vi "Parametric Tester.vi"() -> ()   [LabVIEW 2017]
uses:
  <vilib>/Utility/file.llb/Write To Spreadsheet File (string).vi
  <vilib>/Utility/file.llb/Write To Spreadsheet File (DBL).vi
panel:
  in  "Header Info":string[][](table)=[["Test Name", "Operator", "UUT"], ["Voltage Test", "Nigel", "AAA123"]]
  in  "File Name":path=path "C:/Documents and Settings/husmith/Desktop/CSVdata.csv"
  in  "Channel Names":string[](array[string])=["Channel 1", "Channel 2", "Channel 3", "Channel 4", "Channel 5"]
  in  "# of Channels":i32=5
  in  "stop":bool
  in  "Values to Write":i32=20
  out "Forearm\nAngle":dbl
  out "Backarm\nAngle":dbl
  in  "New Parametric\nValue":dbl
  in  "Points":dbl[][](array[numeric])
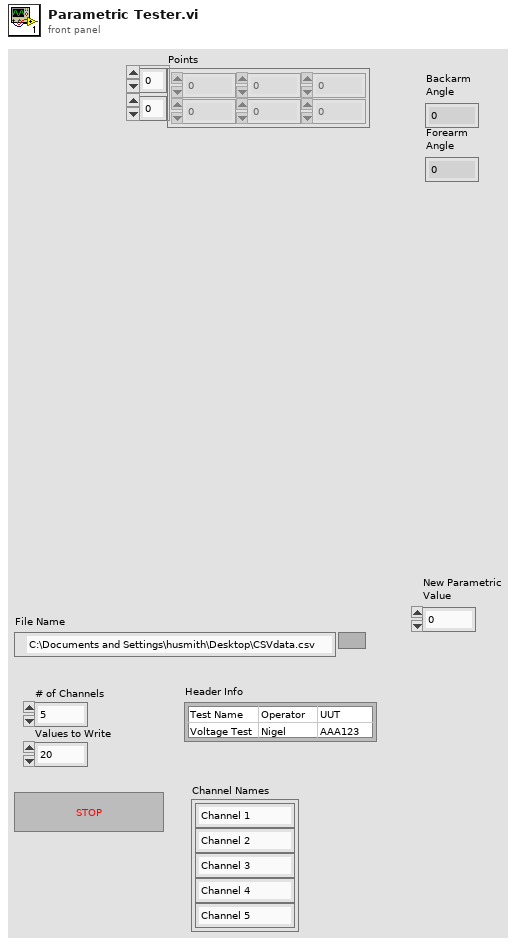
[diagram p1: front panel]
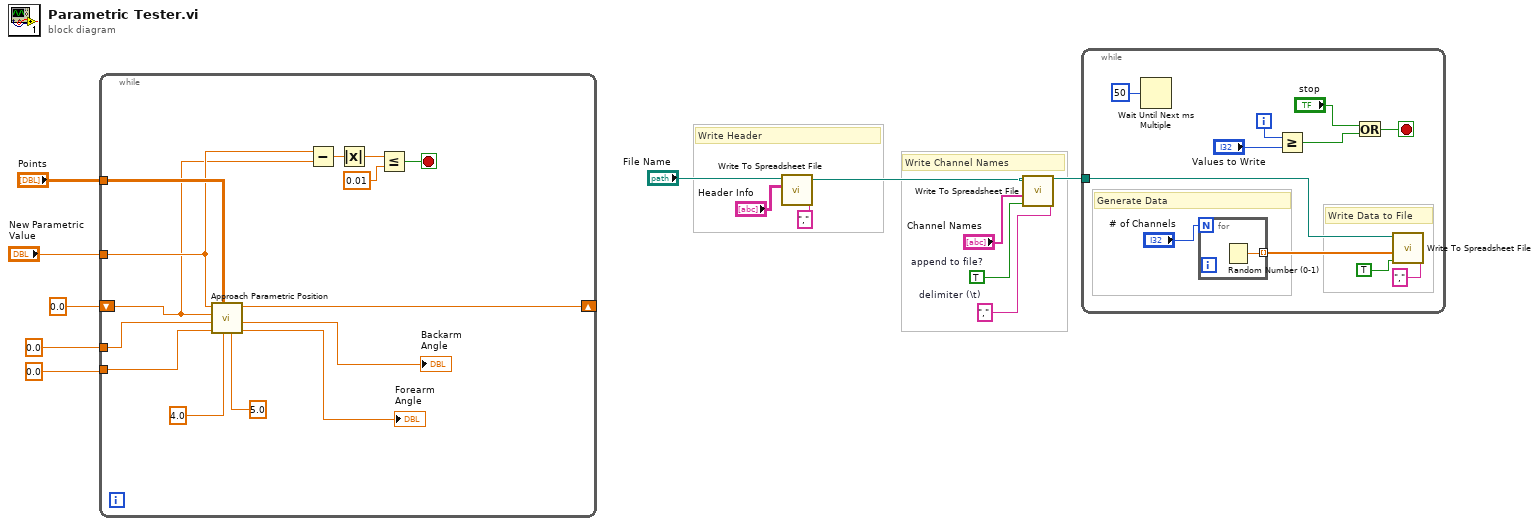
[diagram p0: block diagram]
diagram:
  w4 = TRUE  # append to file?
  w5 = ","  # delimiter (\t)
  # "Write Header"
  # "Write Channel Names"
  n1 = while {
    shift-right: [w23] -> _
    shift-left: 0.0 -> [w20]
    tunnel: "New Parametric\nValue" -> [w21]
    tunnel: 0.0 -> [w27]
    tunnel: 0.0 -> [w26]
    tunnel: "Points" -> [w22]
    stop <- w16 stop-if-true
    n2 = call "Approach Parametric Position.vi"("Forearm Length"=5.0, "Backarm Length"=4.0, "Points"=w22, "Initial Forearm\nAngle"=w26, "Initial Backarm\nAngle"=w27, "Initial Parametric\nValue"=w20, "New Parametric\nValue"=w21) -> ("Next Forearm\nAngle"=→"Forearm\nAngle":dbl, "Next Backarm\nAngle"=→"Backarm\nAngle":dbl, "Next Parametric\nValue"=w23:dbl)  [unwired: 2 in]
    n3 = Subtract(x=w21, y=w20) -> (x-y=w19:dbl)
    n4 = Absolute Value(x=w19) -> (abs(x)=w18:dbl)
    n5 = Less Or Equal?(x=w18, y=0.01) -> (x <= y?=w16:bool)
  }
  n6 = call-poly <vilib>:"Write To Spreadsheet File.vi"("delimiter (\\t)"="," ("delimiter (\\t)"), "2D data"="Header Info", "file path (dialog if empty)"="File Name") -> ("new file path (Not A Path if cancelled)"=w6:path)  [unwired: 4 in, 1 out]
  n7 = call-poly <vilib>:"Write To Spreadsheet File.vi"("delimiter (\\t)"=w5, "append to file? (new file:F)"=w4, "1D data"="Channel Names", "file path (dialog if empty)"=w6) -> ("new file path (Not A Path if cancelled)"=w8:path)  [unwired: 3 in, 1 out]
  n8 = while {
    tunnel: w8 -> [w30]
    i -> [w35]
    stop <- w32 stop-if-true
    # "Write Data to File"
    # "Generate Data"
    n9 = Wait Until Next ms Multiple(millisecond multiple=u32 50) -> ()  [unwired: 1 out]
    n10 = for {
      N: "# of Channels" -> [_]
      tunnel: [w39] -> w31 mode=indexing
      n11 = Random Number (0-1)() -> (number: 0 to 1=w39:dbl)
    }
    n12 = Greater Or Equal?(x=w35, y="Values to Write") -> (x >= y?=w33:bool)
    n13 = Or(x="stop", y=w33) -> (x .or. y?=w32:bool)
    n14 = call-poly <vilib>:"Write To Spreadsheet File.vi"("delimiter (\\t)"="," ("delimiter (\\t)"), "append to file? (new file:F)"=TRUE, "1D data"=w31, "file path (dialog if empty)"=w30) -> ()  [unwired: 3 in, 2 out]
  }
